vi "Untitled 1.vi"() -> ()   [LabVIEW 2018]
panel:
  out "Thermometer":dbl(slide) scale=0.0..100.0
  in  "Numeric":dbl
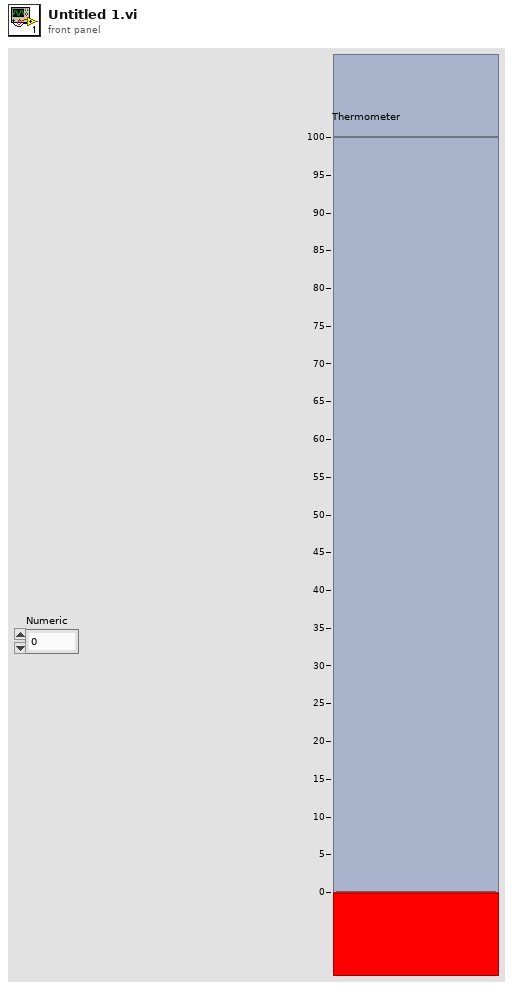
[diagram p1: front panel]
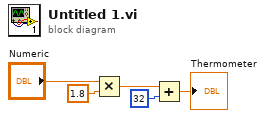
[diagram p0: block diagram]
diagram:
  n1 = Multiply(x="Numeric", y=1.8) -> (x*y=w3:dbl)
  n2 = Add(x=w3, y=32) -> (x+y=→"Thermometer":dbl)
